vi "Create.vi"(8 "error in (no error)":errorcluster, 9 "Group":refnum<class "Group DBL.lvclass">, 10 "Parent Name":string) -> (0 "error out":errorcluster, 3 "Data Logger Module out":refnum<class "Data Logger DBL Module.lvclass">)   [LabVIEW 2020, in "VolatusData.lvlib" / "Data Logger DBL Module.lvclass"]
uses:
  Data Logger DBL Module.lvclass
  lv-vecto/Vecto/Group/Group.lvclass
  lv-vecto/Vecto/Group DBL/Group DBL.lvclass
  C:/dev/lv20CE/relink/lv-vecto/Vecto/Group/Group.lvclass
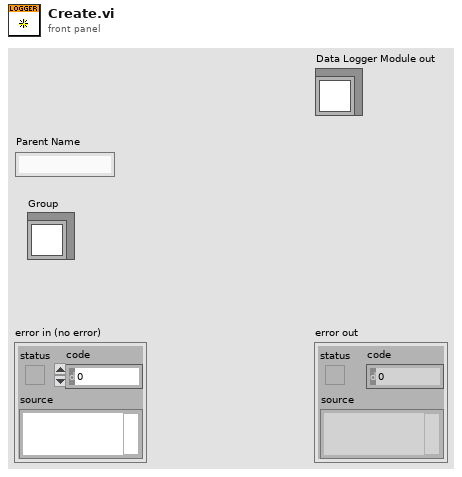
[diagram p1: front panel]
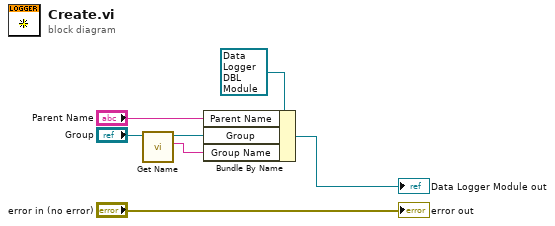
[diagram p0: block diagram]
diagram:
  n1 = call "Get Name.vi"("Group in"="Group") -> ("Name"=w1:string, "Group out"=w2:refnum<class "Group DBL.lvclass">)  [unwired: 8 in, 1 out]
  n2 = Bundle By Name(cluster=refnum<class "Data Logger DBL Module.lvclass"> refnum ("Data Logger Module in"), "Parent Name"="Parent Name", "Group"=w2, "Group Name"=w1) -> (→"Data Logger Module out":refnum<class "Data Logger DBL Module.lvclass">)
  "error out" <- "error in (no error)"
